vi "Configure Debug Data Listener.vi"(8 "error in (no error)":errorcluster, 10 "Debug Data Listener":refnum<class "Debug Data Listener.lvclass">, 11 "Debug Message Receiver In":refnum<class "Debug Message Receiver.lvclass">) -> (0 "error out":errorcluster, 3 "Debug Message Receiver Out":refnum<class "Debug Message Receiver.lvclass">)   [LabVIEW 2020, in "Debug Message Receiver.lvclass"]
uses:
  Debug Message Receiver.lvclass
  C:/Users/anton/Documents/GitHub/triarc-debugger/source/Process/Debug Process.lvclass
  Debug Data Event/Debug Data Listener.lvclass
  Process/Debug Process.lvclass/Debug Process.ctl
  Debug Message Receiver.lvclass/Debug Message Receiver.ctl
  <vilib>/Utility/error.llb/Clear Errors.vi
  <vilib>/Utility/error.llb/Error Cluster From Error Code.vi
  Process/Debug Process.lvclass
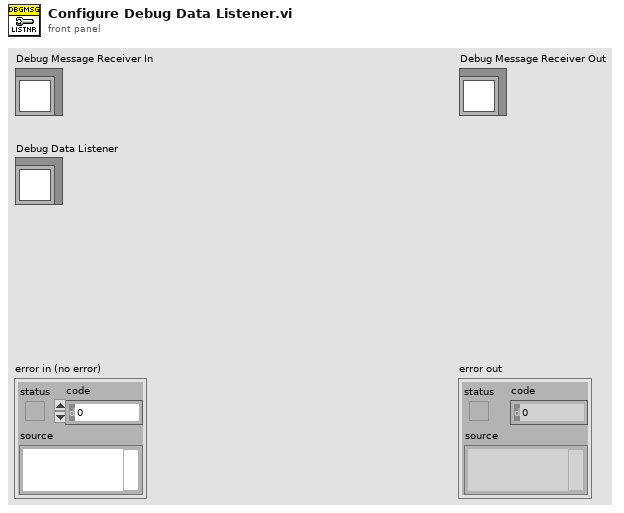
[diagram p1: front panel]
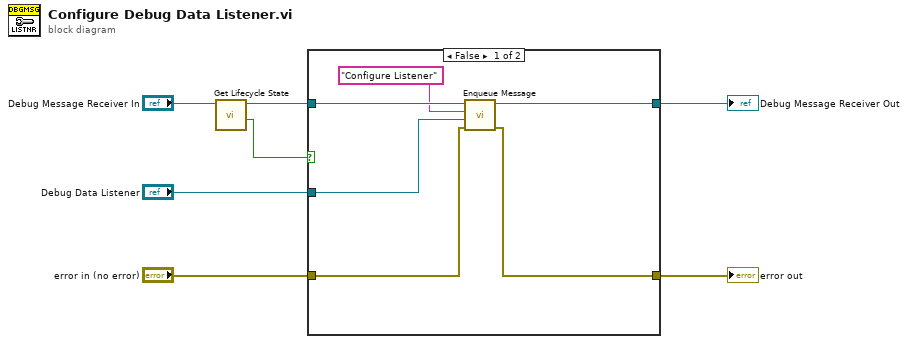
[diagram p0: block diagram]
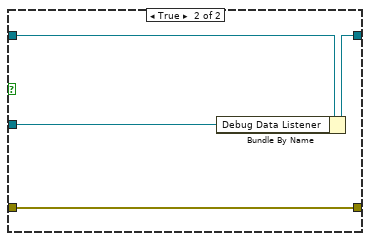
[diagram p2: hidden frame]
diagram:
  n1 = call "Get Lifecycle State.vi"("Process In"="Debug Message Receiver In") -> ("In Process Loop?"=w3:bool, "Process Out"=w4:refnum<class "Debug Message Receiver.lvclass">)  [unwired: 7 in, 2 out]
  n2 = case shown="False" w3 {
    tunnel: [w12 w17] -> w7
    tunnel: "Debug Data Listener" -> [w11 w16]
    tunnel: w4 -> [w13 w15]
    tunnel: "error in (no error)" -> [w10 w14]
    tunnel: [w9 w14] -> w1
    frame False {
      n3 = call "Enqueue Message.vi"("error in (no error)"=w10, "Message Data"=w11, "Message"="Configure Listener", "Process In"=w13) -> ("error out"=w9:errorcluster, "Process Out"=w12:refnum<class "Debug Message Receiver.lvclass">)  [unwired: 6 in]
    }
    frame True {
      n4 = Bundle By Name(cluster=w15, "Debug Data Listener"=w16) -> (w17:refnum<class "Debug Message Receiver.lvclass">)
    }
  }
  "error out" <- w1
  "Debug Message Receiver Out" <- w7
